vi "Main panel.vi"() -> ()   [LabVIEW 2014]
uses:
  C/Program Files/National Instruments/LabVIEW 2014/instr.lib/LeCroy Wave Series/Public/Data/Read Waveform Measurement (Standard).vi
  C/Program Files/National Instruments/LabVIEW 2014/instr.lib/LeCroy Wave Series/LeCroy Wave Series.lvlib
panel:
  out "check f equality":bool
  in  "Reset":bool
  out "wrong f!!":bool
  out "Saving of data":bool caption="Saving Data"
  out "f from osc":dbl
  out "Transfer (dB)":cluster{"Y":dbl[], "Y":dbl[]}[](graph)
  out "f from gen":dbl
  in  "stop":bool
  out "Osc error":errorcluster
  in  "Get values":bool
  in  "Measurement":u16(ring) items=["Amplitude", "Area", "Base", "Cycles", "Delay", "Duration", "Duty Cycle *", "Fall Time (90-10) *", "Fall Time (80-20) *", "First", "Frequency *", "Last", "Maximum", "Mean", "Median", "Minimum", "Num Points", "Overshoot (Negative) *", "Overshoot (Positive) *", "Peak-Peak", "Period *", "Risetime (10-90) *", "Risetime (20-80) *", "RMS", "Standard Deviation", "Top", "Width (Negative slope) *", "Width (Positve slope)"]
  in  "Source / channel":u16(ring) items=["Channel 1", "Channel 2", "Channel 3", "Channel 4", "Memory 1", "Memory 2", "Memory 3", "Memory 4", "Function 1", "Function 2", "Function 3", "Function 4", "Function 5", "Function 6", "Function 7", "Function 8", "Other"]
  in  "Oscilloscope address":refnum<visa-resource-name>
  out "Measured value":dbl
  in  "Offset (V)":dbl min=-5.0 max=5.0 step=0.01
  in  "Output level (V)":dbl min=0.0 max=10.0 step=0.01
  out "f (Hz)":dbl
  in  "index":i32=1 min=1 max=124 step=1
  in  "Setup generator":bool
  in  "Generator address":refnum<visa-resource-name>
  # "Generator setup"
  # "Oscilloscope setup"
  # "Frequency"
  # "Oscilloscope output"
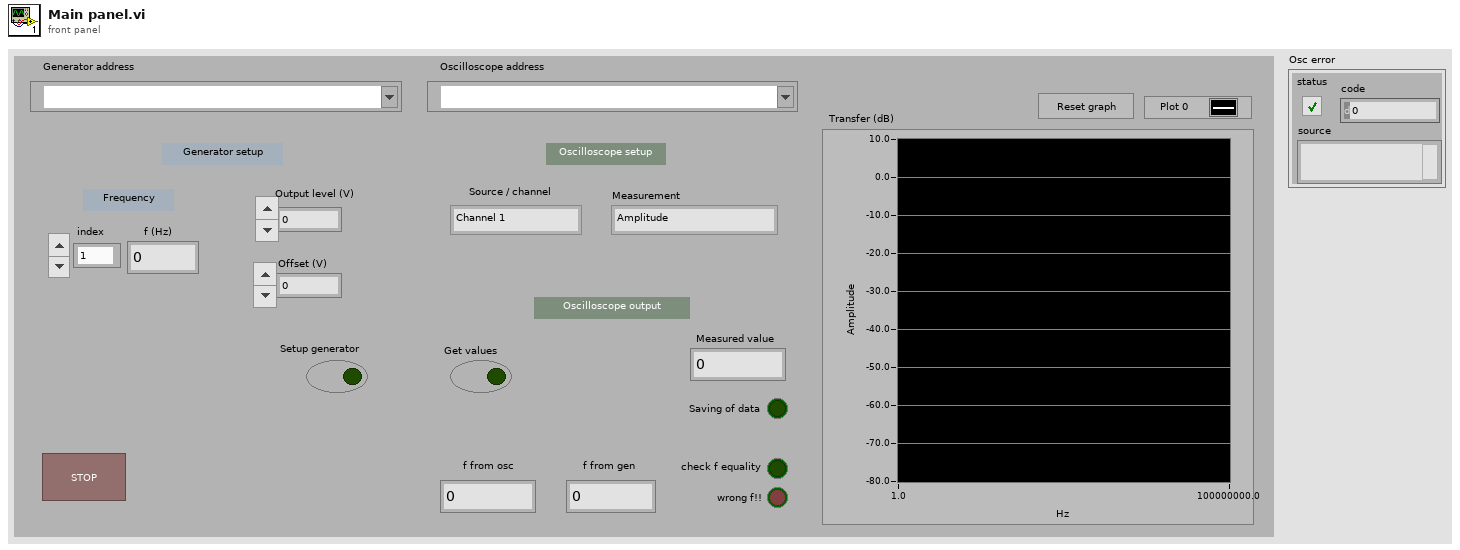
[diagram p1: front panel]
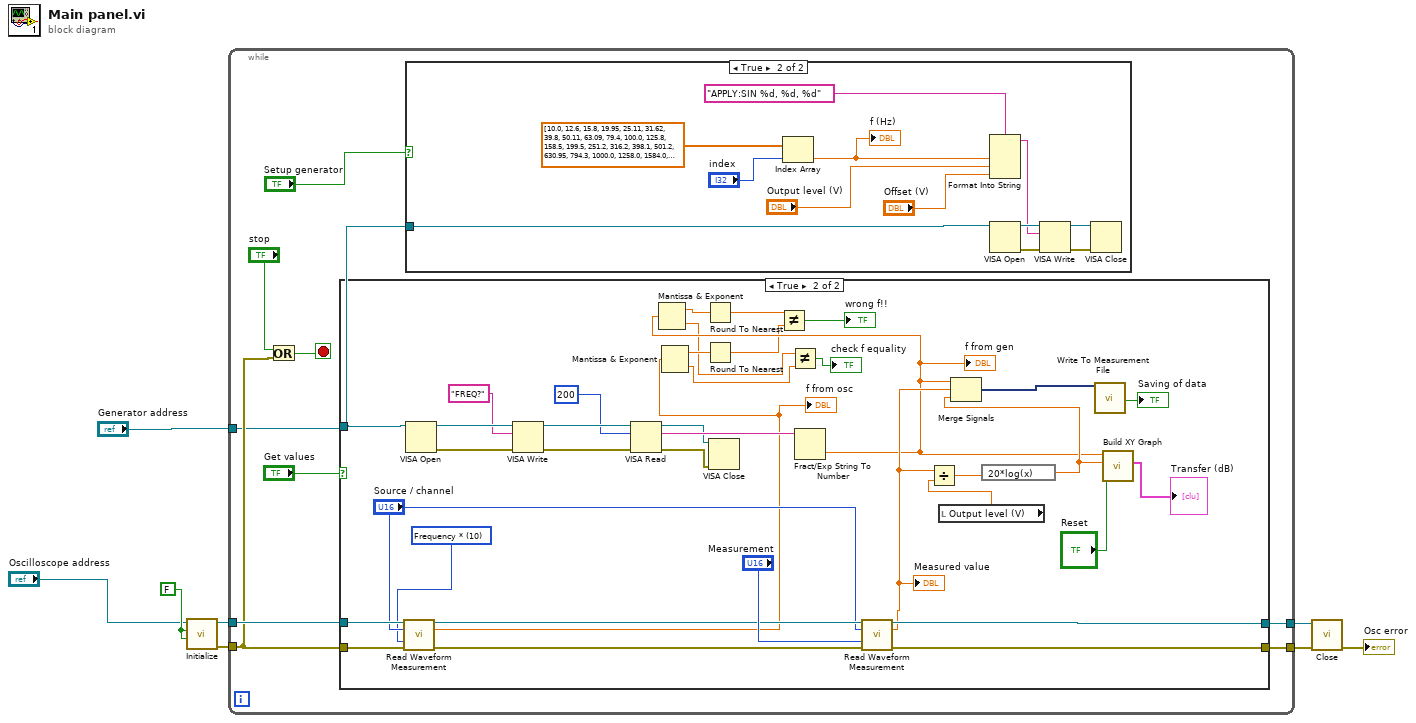
[diagram p0: block diagram]
diagram:
  w5 = FALSE ("Reset? (T: Yes)")
  n1 = call "Initialize.vi"("Reset? (T: Yes)"=w5, "ID Query? (T: Yes)"=w5, "VISA resource name"="Oscilloscope address") -> ("error out"=w2:errorcluster, "VISA resource name out"=w3:refnum<visa-resource-name>)  [unwired: 7 in]
  n2 = while {
    tunnel: [w15] -> w8
    tunnel: [w14] -> w6
    tunnel: w3 -> [w11]
    tunnel: w2 -> [w10]
    tunnel: "Generator address" -> [w9]
    stop <- w13 stop-if-true
    n3 = Or(x="stop", y=w10) -> (x .or. y?=w13:bool)
    n4 = case shown="True" "Get values" {
      tunnel: w11 -> [w19 w38]
      tunnel: w9 -> [_ w56]
      tunnel: [w18 w45] -> w15
      tunnel: w10 -> [w18 w36]
      tunnel: [w19 w44] -> w14
      frame False {
      }
      frame True {
        w33 = u16 10 items=["Amplitude", "Area", "Base", "Cycles", "Delay", "Duration", "Duty Cycle *", "Fall Time (90-10) *", "Fall Time (80-20) *", "First", "Frequency *", "Last", "Maximum", "Mean", "Median", "Minimum", "Num Points", "Overshoot (Negative) *", "Overshoot (Positive) *", "Peak-Peak", "Period *", "Risetime (10-90) *", "Risetime (20-80) *", "RMS", "Standard Deviation", "Top", "Width (Negative slope) *", "Width (Positve slope)"] ("Measurement (0: Amplitude)")
        n5 = call-poly "Read Waveform Measurement.vi"("VISA resource name"=w38, "Source (0: Channel 1)"="Source / channel", "Measurement (0: Amplitude)"=w33, "error in (no error)"=w36) -> ("VISA resource name out"=w37:refnum<visa-resource-name>, "Value"=w29:dbl, "error out"=w35:errorcluster)  [unwired: 8 in, 1 out]
        "f from osc" <- w29
        n6 = VISA Open(VISA resource name=w56) -> (VISA resource name=w55:refnum<visa-resource-name>, error out=w54:errorcluster)  [unwired: 4 in]
        n7 = VISA Write(VISA resource name=w55, write buffer="FREQ?", error in (no error)=w54) -> (VISA resource name out=w52:refnum<visa-resource-name>, error out=w51:errorcluster)  [unwired: 1 out]
        n8 = VISA Read(VISA resource name=w52, byte count=u32 200, error in (no error)=w51) -> (VISA resource name out=w48:refnum<visa-resource-name>, read buffer=w49:string, error out=w47:errorcluster)  [unwired: 1 out]
        n9 = Mantissa & Exponent(0:w29) -> (1:w26:dbl, 2:w22:dbl)
        n10 = Round To Nearest(number=w26) -> (nearest integer value=w24:dbl)
        n11 = VISA Close(VISA resource name=w48, error in (no error)=w47) -> ()  [unwired: 1 out]
        n12 = Fract/Exp String To Number(string=w49) -> (number=w28:dbl)  [unwired: 3 in, 1 out]
        "f from gen" <- w28
        n13 = Mantissa & Exponent(0:w28) -> (1:w27:dbl, 2:w23:dbl)
        n14 = Round To Nearest(number=w27) -> (nearest integer value=w25:dbl)
        n15 = Not Equal?(x=w25, y=w24) -> (x != y?=→"wrong f!!":bool)
        n16 = Not Equal?(x=w23, y=w22) -> (x != y?=→"check f equality":bool)
        n17 = call-poly "Read Waveform Measurement.vi"("VISA resource name"=w37, "Source (0: Channel 1)"="Source / channel", "Measurement (0: Amplitude)"="Measurement", "error in (no error)"=w35) -> ("VISA resource name out"=w44:refnum<visa-resource-name>, "Value"=w39:dbl, "error out"=w45:errorcluster)  [unwired: 8 in, 1 out]
        "Measured value" <- w39
        n18 = local read "Output level (V)"() -> (w41:dbl)
        n19 = Divide(x=w39, y=w41) -> (x/y=w40:dbl)
        n20 = expression code="20*log(x)"(w40) -> (w30:dbl)
        n21 = Merge Signals(w28, w39, w30) -> (w43:dynamicdata)
        n22 = call "Write To Measurement File"("Signals"=w43) -> ("Saving Data"=→"Saving of data":bool)  [unwired: 16 in, 2 out]
        n23 = call "Build XY Graph"("Reset"="Reset", "Y Input"=w30, "X Input"=w28) -> ("XY Graph"=→"Transfer (dB)":cluster{"X":dbl[], "Y":dbl[]}[])  [unwired: 7 in, 1 out]
      }
    }
    n24 = case shown="True" "Setup generator" {
      tunnel: w9 -> [_ w68]
      frame False {
      }
      frame True {
        n25 = Index Array(array=dbl[] [10.0, 12.6, 15.8, 19.95, 25.11, 31.62, 39.8, 50.11, 63.09, 79.4, 100.0, 125.8, 158.5, 199.5, 251.2, 316.2, 398.1, 501.2, 630.95, 794.3, 1000.0, 1258.0, 1584.0, 1995.0, 2511.0, 3162.0, 3981.0, 5012.0, 6309.0, 7943.0, 10000.0, 12589.0, 15848.0, 19952.0, 25118.0, 31622.0, 39810.0, 50118.0, 63095.0, 79432.0, 100000.0, 107977.0, 116591.0, 125892.0, 135935.0, 146779.0, 158489.0, 171132.0, 184785.0, 199526.0, 215443.0, 232630.0, 251188.0, 271227.0, 292864.0, 316227.0, 341454.0, 368694.0, 398107.0, 429866.0, 464158.0, 501187.0, 541169.0, 584341.0, 630957.0, 681292.0, 735642.0, 794328.0, 857698.0, 926118.0, 1000000.0, 1080000.0, 1170000.0, 1260000.0, 1360000.0, 1470000.0, 1580000.0, 1710000.0, 1850000.0, 2000000.0, 2150000.0, 2330000.0, 2510000.0, 2710000.0, 2930000.0, 3160000.0, 3410000.0, 3690000.0, 3980000.0, 4300000.0, 4640000.0, 5010000.0, 5410000.0, 5840000.0, 6310000.0, 6810000.0, 7360000.0, 7940000.0, 8580000.0, 9260000.0, 10000000.0, 10800000.0, 11700000.0, 12600000.0, 13600000.0, 14700000.0, 15800000.0, 17100000.0, 18500000.0, 20000000.0, 21500000.0, 23300000.0, 25100000.0, 27100000.0, 29300000.0, 31600000.0, 34100000.0, 36900000.0, 39800000.0, 43000000.0, 46400000.0, 50100000.0, 54100000.0, 58400000.0, 60000000.0], index="index") -> (element=w64:dbl)
        "f (Hz)" <- w64
        n26 = Format Into String(format string="APPLY:SIN %d, %d, %d", w64, "Output level (V)", "Offset (V)") -> (resulting string=w60:string)  [unwired: 2 in, 1 out]
        n27 = VISA Open(VISA resource name=w68) -> (VISA resource name=w67:refnum<visa-resource-name>, error out=w59:errorcluster)  [unwired: 4 in]
        n28 = VISA Write(VISA resource name=w67, write buffer=w60, error in (no error)=w59) -> (VISA resource name out=w57:refnum<visa-resource-name>, error out=w58:errorcluster)  [unwired: 1 out]
        n29 = VISA Close(VISA resource name=w57, error in (no error)=w58) -> ()  [unwired: 1 out]
      }
    }
  }
  n30 = call "Close.vi"("error in (no error)"=w8, "VISA resource name"=w6) -> ("error out"=→"Osc error":errorcluster)  [unwired: 9 in]
